vi "has params.vi"(8 "error in (no error)":errorcluster, 11 "Request in":refnum<class "Request.lvclass">) -> (0 "error out":errorcluster, 2 "has params?":bool, 3 "Request out":refnum<class "Request.lvclass">)   [LabVIEW 2016, in "Request.lvclass"]
uses:
  Request.lvclass
  <vilib>/NI/JSON Support for LabVIEW/JSON Types.ctl
  Request.lvclass/Request.ctl
  <vilib>/NI/JSON Support for LabVIEW/JSON Data Classes/JSON Datatype/JSON Null.lvclass
  <vilib>/NI/JSON Support for LabVIEW/LVJSON.lvlib
  params/params.lvclass
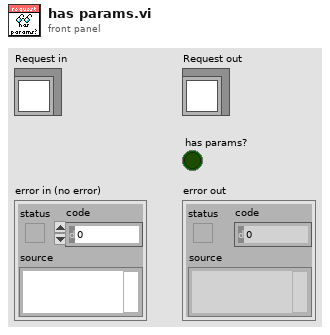
[diagram p1: front panel]
types:
  T1 = typedef "LVJSON.lvlib/JSON Types.ctl" = enum16{"String", "Numeric", "Boolean", "NULL", "Object", "Array"}
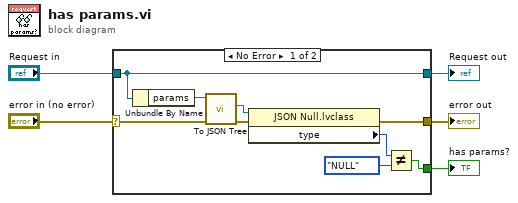
[diagram p0: block diagram]
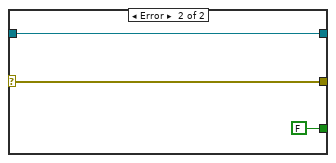
[diagram p2: hidden frame]
diagram:
  n1 = case shown="No Error" "error in (no error)" {
    selector: "error in (no error)" -> [w8 w17]
    tunnel: [w6 w17] -> w4
    tunnel: [w14 w16] -> w2
    tunnel: "Request in" -> [w14 w16]
    tunnel: [w13 FALSE] -> w1
    frame No Error {
      n2 = Unbundle By Name(w14) -> ("params"=w12:refnum<class "params.lvclass">)
      n3 = call "To JSON Tree.vi"("error in (no error)"=w8, "params in"=w12) -> ("error out"=w7:errorcluster, "JSON out"=w11:refnum<class "JSON Null.lvclass">)  [unwired: 7 in, 1 out]
      n4 = property class="JSON Null.lvclass"(reference=w11, error in=w7) -> (error out=w6:errorcluster, "type"=w10:T1)  [unwired: 1 out]
      n5 = Not Equal?(x=w10, y=JSON_Types."NULL" ("type")) -> (x != y?=w13:bool)
    }
    frame Error {
    }
  }
  "error out" <- w4
  "Request out" <- w2
  "has params?" <- w1
